vi "Lift Control.vi"(10 "MotorControlDevRefLeft":T2={"DeviceStatus"={"status"=FALSE, "code"=0, "source"=""}, "Type"=enum."PWM", "PWM"={"PWM Channel"=enum."Invalid", "DeadBand"={"Name"="", "maxPositivePwm"=0, "minPositivePwm"=0, "centerPwm"=0, "maxNegativePwm"=0, "minNegativePwm"=0, "angularRange"=0}}, "CAN"={"Device Number"=0, "Control Mode"=enum."Percent VBus", "Semaphore"=refnum, "Max Vout"=12.0, "TalonSRX Control Mode"=enum."Percent VBus"}, "Invert"=FALSE}, 11 "MotorControlDevRefRight":T2={"DeviceStatus"={"status"=FALSE, "code"=0, "source"=""}, "Type"=enum."PWM", "PWM"={"PWM Channel"=enum."Invalid", "DeadBand"={"Name"="", "maxPositivePwm"=0, "minPositivePwm"=0, "centerPwm"=0, "maxNegativePwm"=0, "minNegativePwm"=0, "angularRange"=0}}, "CAN"={"Device Number"=0, "Control Mode"=enum."Percent VBus", "Semaphore"=refnum, "Max Vout"=12.0, "TalonSRX Control Mode"=enum."Percent VBus"}, "Invert"=FALSE}) -> ()   [LabVIEW 2015]
doc: "Controls the lift system from global variables."
uses:
  <vilib>/Rock Robotics/WPI/MotorControl/WPI_MotorControlDeviceRef.ctl
  <vilib>/Rock Robotics/WPI/MotorControl/WPI_MotorControlType.ctl
  <vilib>/Rock Robotics/SystemInterfaces/DIO/FPGA_DIOPWMChannel.ctl
  <vilib>/Rock Robotics/WPI/PWM/WPI_PWMDeadband.ctl
  <vilib>/Rock Robotics/WPI/CAN/Jaguar/SubVIs/WPI_CANJaguar_ControlMode.ctl
  <vilib>/Rock Robotics/WPI/CAN/TalonSRX/WPI_CANTalonSRX_APIControlMode.ctl
  <vilib>/Rock Robotics/WPI/DriverStation/WPI_DriverStationRobotMode2.ctl
  <vilib>/Analysis/3filter.llb/Filter Passband Type.ctl
  Robot Values.vi
  Robot Global Data.vi
  <vilib>/addons/control/pid/pid.llb/PID (DBL).vi
  <vilib>/addons/control/pid/NI_PID_pid.lvlib
  <vilib>/ptbypt/NI_PtbyPt.lvlib
  <vilib>/Analysis/NI_AALBase.lvlib
panel:
  out "Waveform Chart":dbl(graph)
  out "Overridelasthieght":dbl format="%#_13g"
  in  "initialize":bool
  in  "Manual gains":T1={"proportional gain (Kc)"=0.08, "integral time (Ti, min)"=0.0, "derivative time (Td, min)"=0.0} {"derivative time (Td, min)" format="%.3f"; "integral time (Ti, min)" format="%.3f"; "proportional gain (Kc)" format="%.3f"}
  in  "low cutoff freq: fl":dbl=0.08 format="%#_13g"
  in  "Diffrence gains":T1={"proportional gain (Kc)"=0.08, "integral time (Ti, min)"=0.0, "derivative time (Td, min)"=0.0} {"derivative time (Td, min)" format="%.3f"; "integral time (Ti, min)" format="%.3f"; "proportional gain (Kc)" format="%.3f"}
  in  "Average gains":T1={"proportional gain (Kc)"=0.1, "integral time (Ti, min)"=0.0, "derivative time (Td, min)"=0.001} {"derivative time (Td, min)" format="%.3f"; "integral time (Ti, min)" format="%.4f"; "proportional gain (Kc)" format="%.3f"}
  in  "Left encoder offset":dbl=0.5 format="%#_13g"
  in  "motor Deadband":dbl=0.05
  in  "Desired Heights":dbl[](array[numeric])=[0.0, 21.5, 77.5, 110.0]
  in  "PID Gains":T1={"proportional gain (Kc)"=0.02, "integral time (Ti, min)"=0.0009999999999999992, "derivative time (Td, min)"=0.001} {"derivative time (Td, min)" format="%.3f"; "integral time (Ti, min)" format="%.3f"; "proportional gain (Kc)" format="%.3f"}
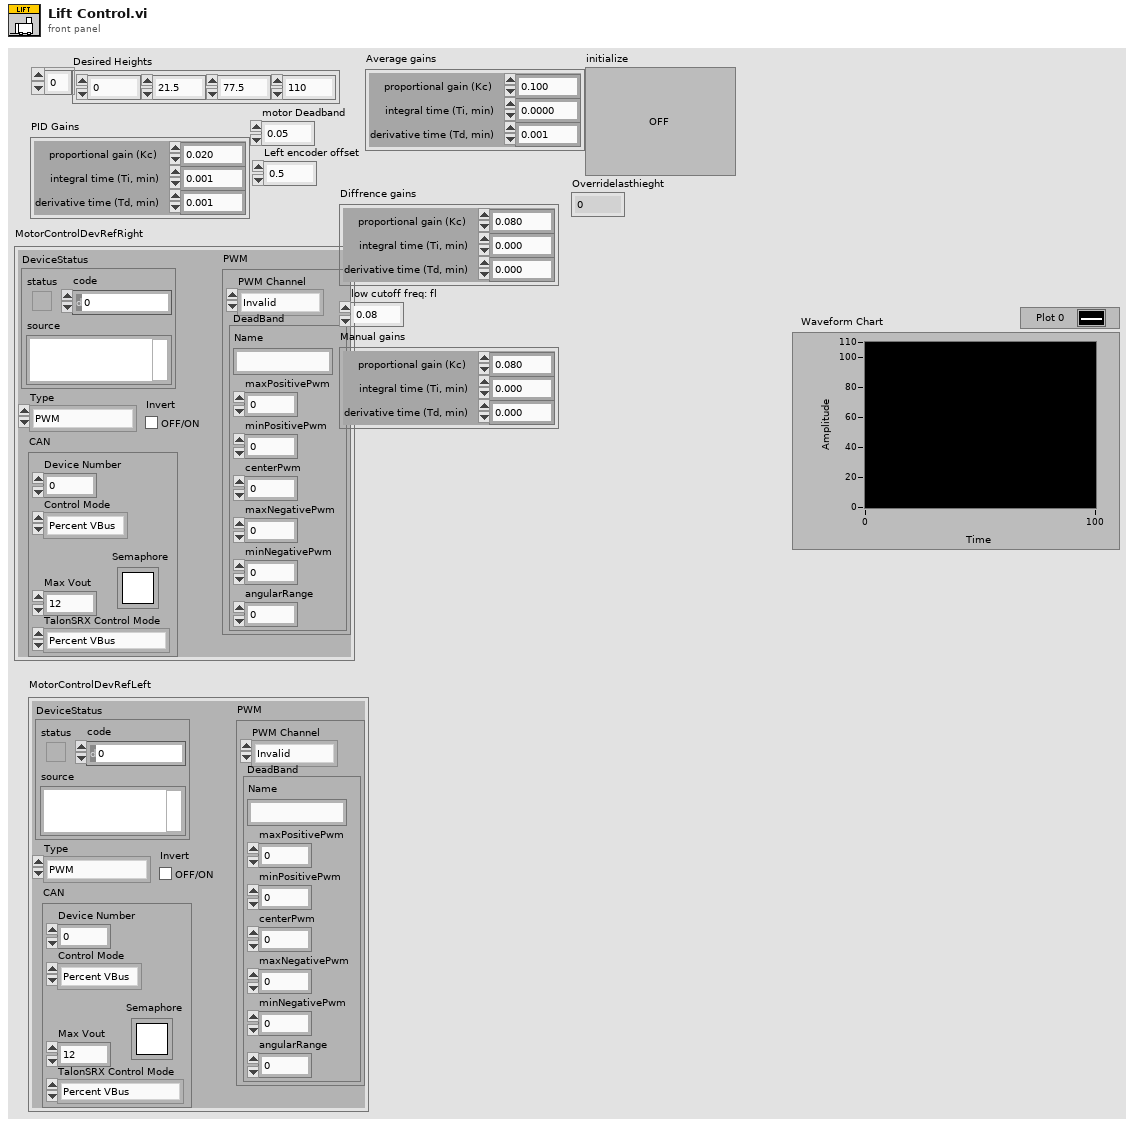
[diagram p1: front panel]
types:
  T1 = cluster{"proportional gain (Kc)":dbl, "integral time (Ti, min)":dbl, "derivative time (Td, min)":dbl}
  T2 = typedef "WPI_MotorControlDeviceRef.ctl" = cluster{"DeviceStatus":errorcluster, "Type":T3, "PWM":cluster{"PWM Channel":T4, "DeadBand":T5}, "CAN":cluster{"Device Number":u8, "Control Mode":T6, "Semaphore":T7, "Max Vout":dbl, "TalonSRX Control Mode":T8}, "Invert":bool}
  T3 = typedef "WPI_MotorControlType.ctl" = enum16{"PWM", "CAN", "CANTalonSRX"}
  T4 = typedef "FPGA_DIOPWMChannel.ctl" = enum8{"PWM 0", "PWM 1", "PWM 2", "PWM 3", "PWM 4", "PWM 5", "PWM 6", "PWM 7", "PWM 8", "PWM 9", "PWM MXP 0", "PWM MXP 1", "PWM MXP 2", "PWM MXP 3", "PWM MXP 4", "PWM MXP 5", "PWM MXP 6", "PWM MXP 7", "PWM MXP 8", "PWM MXP 9", "Invalid"}
  T5 = typedef "WPI_PWMDeadband.ctl" = cluster{"Name":string, "maxPositivePwm":i32, "minPositivePwm":i32, "centerPwm":i32, "maxNegativePwm":i32, "minNegativePwm":i32, "angularRange":u16}
  T6 = typedef "WPI_CANJaguar_ControlMode.ctl" = enum8{"Percent VBus", "Current", "Speed", "Position", "Voltage"}
  T7 = typedef "Semaphore RefNum" = refnum<k1>
  T8 = typedef "WPI_CANTalonSRX_APIControlMode.ctl" = enum8{"Percent VBus", "Speed", "Position", "Slave", "Unchanged / Invalid", "Voltage Compensation", "Current", "Motion Profile"}
  T9 = typedef "NI_AALBase.lvlib/Filter Passband Type.ctl" = enum32{"Lowpass", "Highpass", "Bandpass", "Bandstop"}
  T10 = typedef "WPI_DriverStationRobotMode2.ctl" = enum16{"Autonomous Disabled", "Autonomous Enabled", "Teleop Disabled", "Teleop Enabled", "Disconnected", "Finish", "Test Disabled", "Test Enabled", "Emergency Stopped"}
  T11 = cluster{"Lift Position":i32, "Lift Speed Override":dbl, "OverrideTele?":bool, "OverrideDash":bool}
  T12 = cluster{"Lift Encoder Height Right (cm)":dbl, "Lift Encoder Height Left (cm)":dbl, "Right Prox":bool, "Left Prox":bool, "Gyro Angle":dbl, "Gyro anglar rate":dbl, "Gyro Reset":bool, "Drive encoder Dash reset":bool}
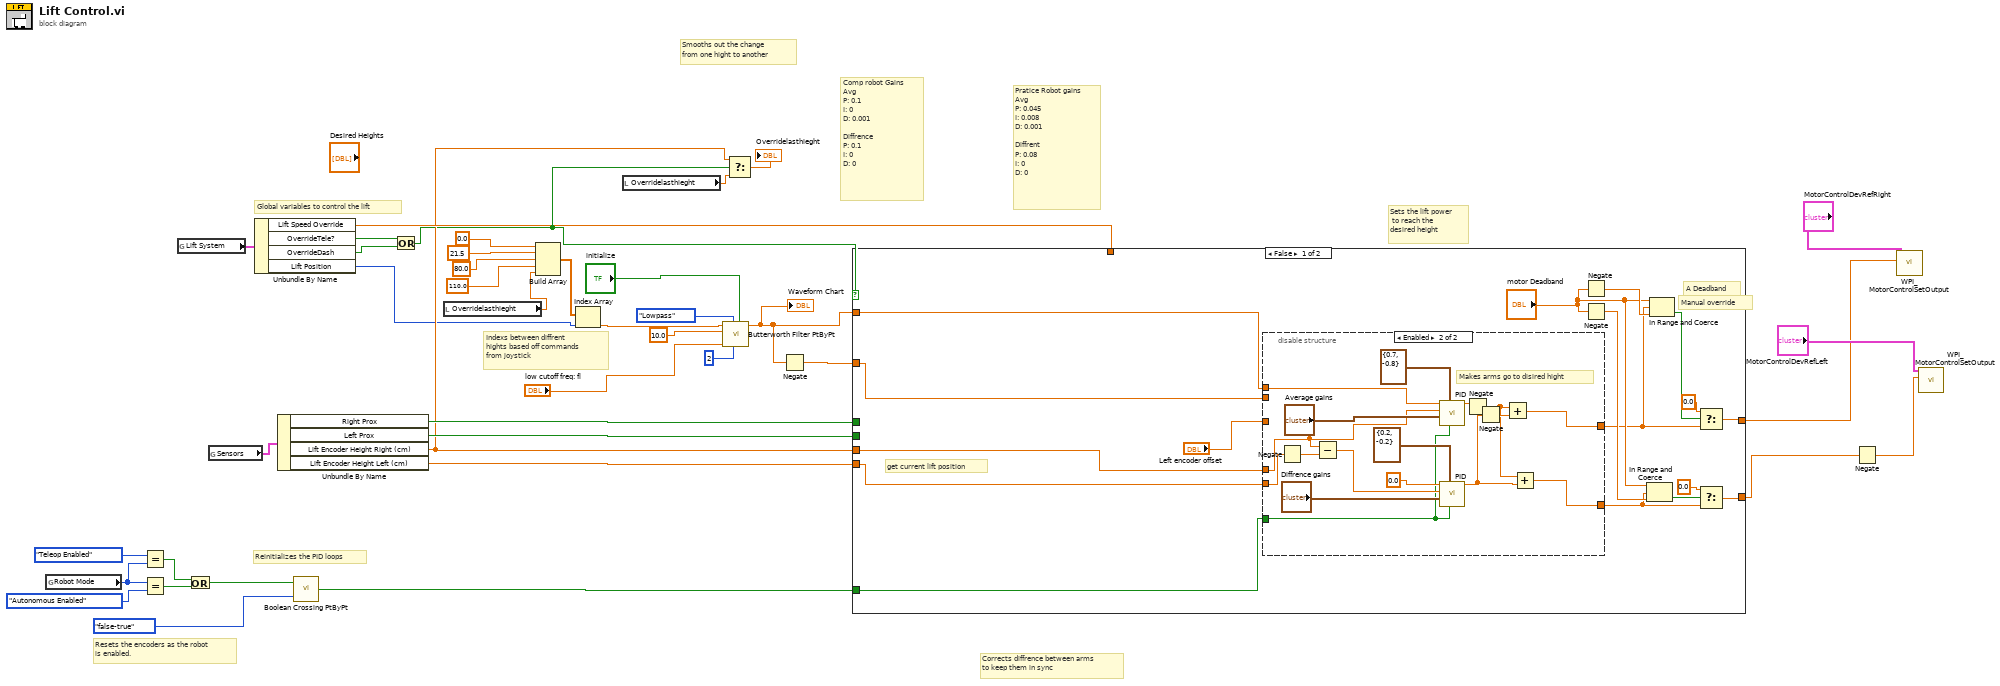
[diagram p0: block diagram]
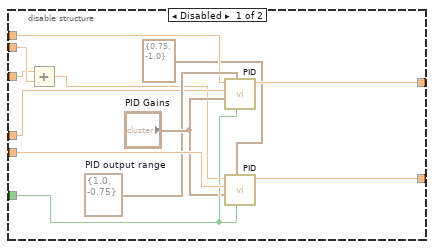
[diagram p2: hidden frame]
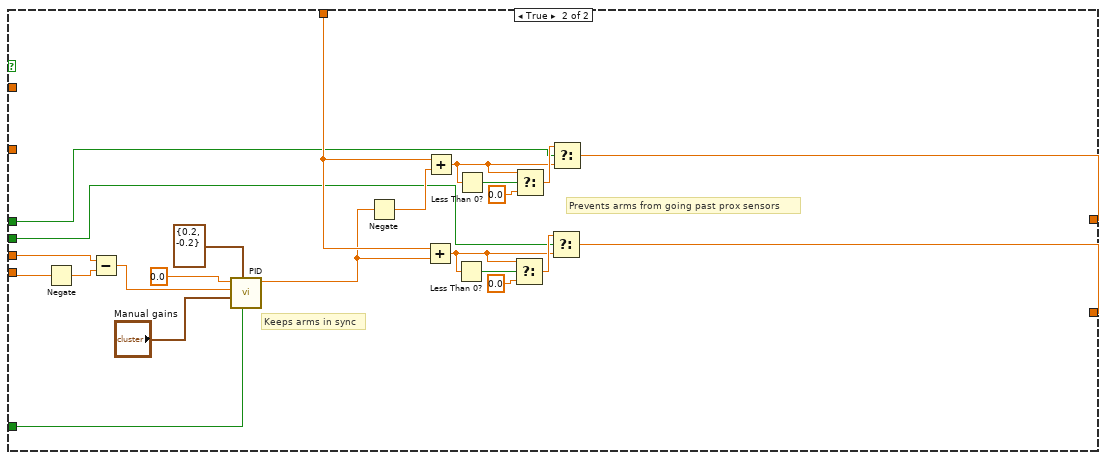
[diagram p3: hidden frame]
diagram:
  # "Indexs between diffrent\nhights based off commands\nfrom joystick"
  # "Smooths out the change\nfrom one hight to another"
  # "Pratice Robot gains\nAvg\nP: 0.045\nI: 0.008\nD: 0.001\n\nDiffrent\nP: 0.08\nI: 0\nD: 0"
  # "Comp robot Gains\nAvg\nP: 0.1\nI: 0\nD: 0.001\n\nDiffrence\nP: 0.1\nI: 0\nD: 0"
  # "Corrects diffrence between arms\nto keep them in sync"
  # "Reinitializes the PID loops"
  # "Resets the encoders as the robot\nis enabled."
  # "Global variables to control the lift"
  # "Manual override"
  # "Sets the lift power\n to reach the \ndesired height"
  n1 = global read "Robot Global Data.vi" "Robot Mode"() -> (w28:T10)
  n2 = Equal?(x=WPI_DriverStationRobotMode2."Teleop Enabled" ("y"), y=w28) -> (x = y?=w25:bool)
  n3 = Equal?(x=w28, y=WPI_DriverStationRobotMode2."Autonomous Enabled") -> (x = y?=w26:bool)
  n4 = global read "Robot Values.vi" "Lift System"() -> (w39:T11)
  n5 = Or(x=w25, y=w26) -> (x .or. y?=w27:bool)
  n6 = global read "Robot Values.vi" "Sensors"() -> (w32:T12)
  n7 = Unbundle By Name(w39) -> ("Lift Speed Override"=w30:dbl, "OverrideTele?"=w36:bool, "OverrideDash"=w35:bool, "Lift Position"=w4:i32)
  n8 = Unbundle By Name(w32) -> ("Right Prox"=w21:bool, "Left Prox"=w20:bool, "Lift Encoder Height Right (cm)"=w17:dbl, "Lift Encoder Height Left (cm)"=w31:dbl)
  n9 = call <vilib>:"Boolean Crossing PtByPt.vi"("direction"=enum16{"either", "false-true", "true-false"}."false-true", "input"=w27) -> ("crossing"=w22:bool)  [unwired: 1 in]
  n10 = Or(x=w36, y=w35) -> (x .or. y?=w2:bool)
  n11 = local read "Overridelasthieght"() -> (w14:dbl)
  n12 = Build Array(0.0 ("element"), 21.5 ("element"), 80.0 ("element"), 110.0 ("element"), w14) -> (w15:dbl[])
  n13 = Index Array(array=w15, index=w4) -> (element=w16:dbl)
  n14 = local read "Overridelasthieght"() -> (w18:dbl)
  n15 = call <vilib>:"Butterworth Filter PtByPt.vi"("initialize"="initialize", "order"=2, "filter type"=Filter_Passband_Type."Lowpass", "low cutoff freq: fl"="low cutoff freq: fl", "sampling freq: fs"=10.0, "x"=w16) -> ("Filtered x"=w3:dbl)  [unwired: 3 in, 1 out]
  "Waveform Chart" <- w3
  n16 = Select(t=w17, s=w2, f=w18) -> (s? t:f=→"Overridelasthieght":dbl)
  n17 = Negate(x=w3) -> (-x=w5:dbl)
  n18 = case shown="False" w2 {
    tunnel: [w47 w87] -> w34
    tunnel: [w44 w98] -> w33
    tunnel: w17 -> [w43 w107]
    tunnel: w31 -> [w46 w109]
    tunnel: w30 -> [_ w102]
    tunnel: w22 -> [w45 w101]
    tunnel: w21 -> [_ w89]
    tunnel: w20 -> [_ w88]
    tunnel: w3 -> [w42 _]
    tunnel: w5 -> [w41 _]
    frame False {
      # "A Deadband"
      # "get current lift position"
      n19 = disable-structure shown="Enabled" {
        disable-tunnel: w46 -> [w69 w85]
        disable-tunnel: w45 -> [w68 w76]
        disable-tunnel: w43 -> [w65 w77]
        disable-tunnel: [w64 w74] -> w50
        disable-tunnel: [w63 w75] -> w49
        disable-tunnel: w42 -> [w62 w86]
        disable-tunnel: w41 -> [w60 _]
        disable-tunnel: "Left encoder offset" -> [w59 _]
        frame Disabled {
          w66 = cluster{"output high":dbl, "output low":dbl} {"output high"=1.0, "output low"=-0.75}  # PID output range
          n20 = Add(x=w59, y=w60) -> (x+y=w58:dbl)
          n21 = call-poly <vilib>:"PID.vi"("reinitialize? (F)"=w68, "output range"=w66, "PID gains"="PID Gains", "process variable"=w65, "setpoint"=w62) -> ("output"=w64:dbl)  [unwired: 5 in, 1 out]
          n22 = call-poly <vilib>:"PID.vi"("reinitialize? (F)"=w68, "output range"=cluster{"output high":dbl, "output low":dbl} {"output high"=0.75, "output low"=-1.0}, "PID gains"="PID Gains", "process variable"=w69, "setpoint"=w58) -> ("output"=w63:dbl)  [unwired: 5 in, 1 out]
        }
        frame Enabled {
          # "Makes arms go to disired hight"
          n23 = Negate(x=w85) -> (-x=w82:dbl)
          n24 = Subtract(x=w77, y=w82) -> (x-y=w81:dbl)
          n25 = call-poly <vilib>:"PID.vi"("reinitialize? (F)"=w76, "output range"=cluster{"output high":dbl, "output low":dbl} {"output high"=0.7, "output low"=-0.8}, "PID gains"="Average gains", "process variable"=w77, "setpoint"=w86) -> ("output"=w73:dbl)  [unwired: 5 in, 1 out]
          n26 = call-poly <vilib>:"PID.vi"("reinitialize? (F)"=w76, "output range"=cluster{"output high":dbl, "output low":dbl} {"output high"=0.2, "output low"=-0.2}, "PID gains"="Diffrence gains", "process variable"=w81, "setpoint"=0.0) -> ("output"=w72:dbl)  [unwired: 5 in, 1 out]
          n27 = Negate(x=w73) -> (-x=w70:dbl)
          n28 = Negate(x=w72) -> (-x=w71:dbl)
          n29 = Add(x=w70, y=w71) -> (x+y=w74:dbl)
          n30 = Add(x=w70, y=w72) -> (x+y=w75:dbl)
        }
      }
      n31 = Negate(x="motor Deadband") -> (-x=w54:dbl)
      n32 = Negate(x="motor Deadband") -> (-x=w57:dbl)
      n33 = In Range and Coerce(upper limit="motor Deadband", x=w49, lower limit=w57) -> (In Range?=w56:bool)  [unwired: 1 out]
      n34 = In Range and Coerce(upper limit="motor Deadband", x=w50, lower limit=w54) -> (In Range?=w53:bool)  [unwired: 1 out]
      n35 = Select(t=0.0, s=w53, f=w50) -> (s? t:f=w44:dbl)
      n36 = Select(t=0.0, s=w56, f=w49) -> (s? t:f=w47:dbl)
    }
    frame True {
      # "Prevents arms from going past prox sensors"
      # "Keeps arms in sync"
      n37 = Negate(x=w109) -> (-x=w108:dbl)
      n38 = Subtract(x=w107, y=w108) -> (x-y=w106:dbl)
      n39 = call-poly <vilib>:"PID.vi"("reinitialize? (F)"=w101, "output range"=cluster{"output high":dbl, "output low":dbl} {"output high"=0.2, "output low"=-0.2}, "PID gains"="Manual gains", "process variable"=w106, "setpoint"=0.0) -> ("output"=w100:dbl)  [unwired: 5 in, 1 out]
      n40 = Negate(x=w100) -> (-x=w99:dbl)
      n41 = Add(x=w102, y=w100) -> (x+y=w90:dbl)
      n42 = Add(x=w102, y=w99) -> (x+y=w94:dbl)
      n43 = Less Than 0?(x=w90) -> (x < 0?=w92:bool)
      n44 = Less Than 0?(x=w94) -> (x < 0?=w96:bool)
      n45 = Select(t=w90, s=w92, f=0.0) -> (s? t:f=w93:dbl)
      n46 = Select(t=w94, s=w96, f=0.0) -> (s? t:f=w97:dbl)
      n47 = Select(t=w93, s=w88, f=w90) -> (s? t:f=w87:dbl)
      n48 = Select(t=w97, s=w89, f=w94) -> (s? t:f=w98:dbl)
    }
  }
  n49 = Negate(x=w34) -> (-x=w37:dbl)
  n50 = call <vilib>:"WPI_MotorControlSetOutput.vi"("Output"=w33, "MotorControlDevRef"="MotorControlDevRefRight") -> ()  [unwired: 7 in, 3 out]
  n51 = call <vilib>:"WPI_MotorControlSetOutput.vi"("Output"=w37, "MotorControlDevRef"="MotorControlDevRefLeft") -> ()  [unwired: 7 in, 3 out]
